vi "replace shared memory file string.vi"(9 "new string":string="MeMeMe", 10 "file name":string="EngineName_input_Double_You") -> (2 "new file name":string)   [LabVIEW 2013, in "Shared Memory editor node.lvclass"]
uses:
  Shared Memory editor node.lvclass
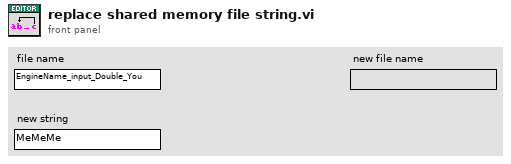
[diagram p1: front panel]
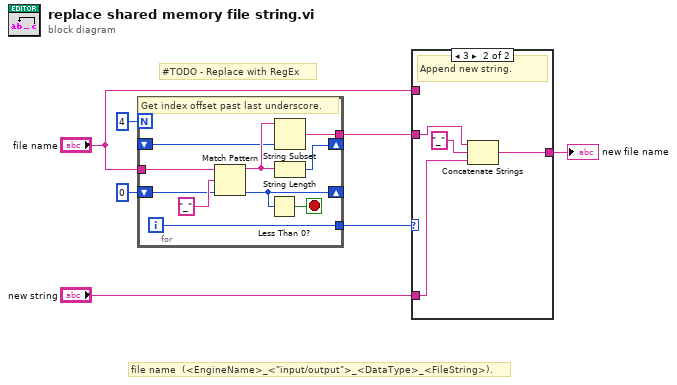
[diagram p0: block diagram]
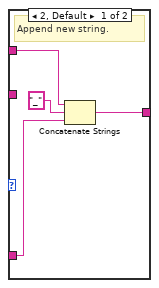
[diagram p2: hidden frame]
diagram:
  # "file name  (<EngineName>_<\"input/output\">_<DataType>_<FileString>)."
  # "#TODO - Replace with RegEx"
  n1 = for {
    N: 4 -> [_]
    shift-right: [w15] -> _
    shift-left: 0 ("offset past match") -> [w13]
    tunnel: "file name" -> [w17]
    tunnel: [w12] -> w5
    shift-right: [w11] -> _
    shift-left: _ -> [w9]
    tunnel: [w8] -> w1
    i -> [w12]
    stop <- w14 stop-if-true
    # "Get index offset past last underscore."
    n2 = Match Pattern(string=w17, regular expression="_", offset (0)=w13) -> (before substring=w10:string, offset past match=w15:i32)  [unwired: 2 out]
    n3 = Less Than 0?(x=w15) -> (x < 0?=w14:bool)
    n4 = String Subset(string=w10, length (rest)=w9) -> (substring=w8:string)  [unwired: 1 in]
    n5 = String Length(string=w10) -> (length=w11:i32)
  }
  n6 = case shown="3" w5 {
    tunnel: "new string" -> [w21 w25]
    tunnel: [w20 w24] -> w3
    tunnel: "file name" -> [w19 _]
    tunnel: w1 -> [_ w22]
    frame 2, Default {
      # "Append new string."
      n7 = Concatenate Strings(w19, "_" ("regular expression"), w21) -> (w20:string)
    }
    frame 3 {
      # "Append new string."
      n8 = Concatenate Strings(w22, "_" ("regular expression"), w25) -> (w24:string)
    }
  }
  "new file name" <- w3
